vi "F to C converter.vi"(1 "Convert":dbl) -> ()   [LabVIEW 2013]
panel:
  in  "milliseconds to wait":u32(slide) scale=0.0..1000.0
  out "System Waveform Graph":dbl[](graph)
  out "Waveform Graph":dbl[](graph)
  out "Numeric":dbl
  out "Waveform Chart":dbl(graph)
  in  "stop":bool
  in  "Temperature (F)":dbl(slide) scale=0.0..212.0
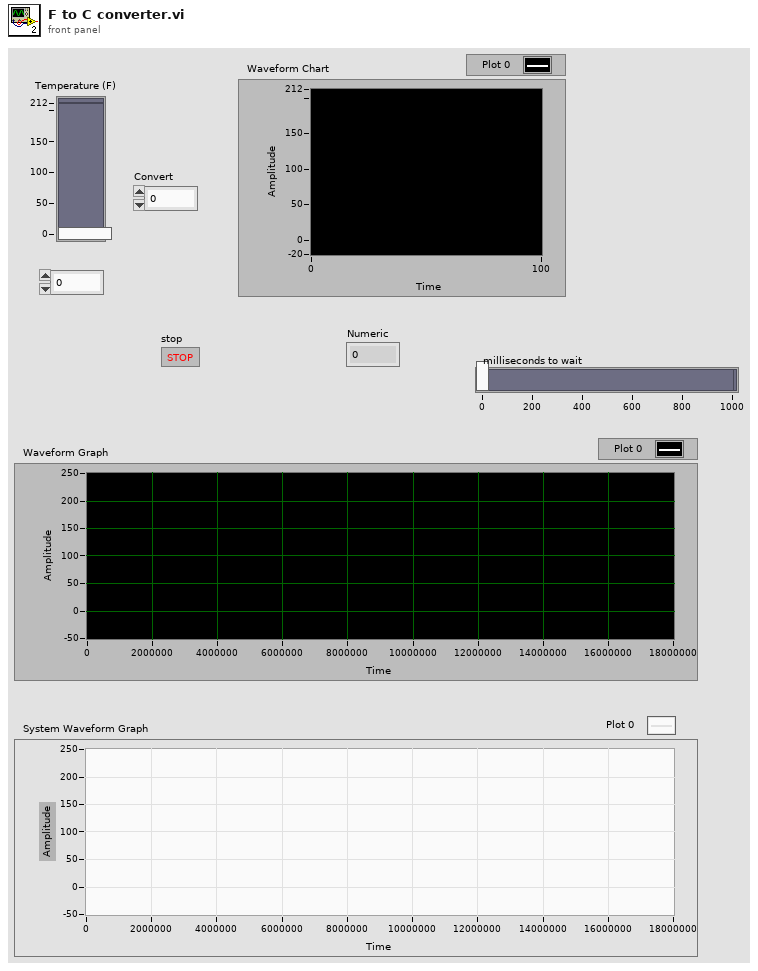
[diagram p1: front panel]
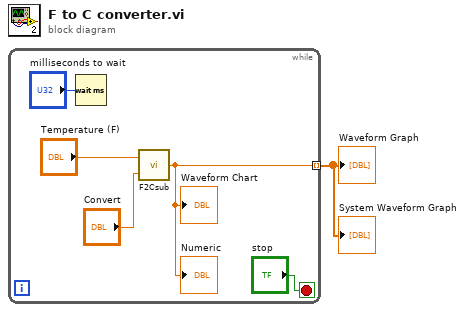
[diagram p0: block diagram]
diagram:
  n1 = while {
    tunnel: [w3] -> w1 mode=indexing
    stop <- "stop" stop-if-true
    n2 = Wait (ms)(milliseconds to wait="milliseconds to wait") -> ()  [unwired: 1 out]
    n3 = call "F2Csub.vi"("Numeric 2"="Convert", "Temperature (F)"="Temperature (F)") -> ("Numeric"=w3:dbl)
    "Waveform Chart" <- w3
    "Numeric" <- w3
  }
  "Waveform Graph" <- w1
  "System Waveform Graph" <- w1
